vi "启动日志.vi"(8 "error in (no error)":errorcluster, 10 "日志信息":string, 11 "Slave ID":T1=enum."氨氮") -> (0 "error out":errorcluster)   [LabVIEW 2016, in "质控单元V1.lvlib"]
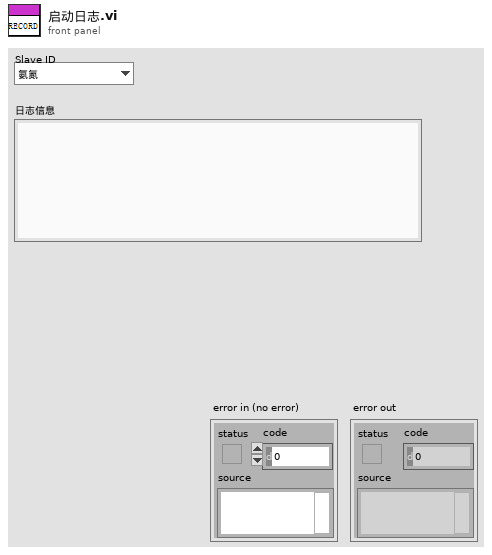
[diagram p1: front panel]
types:
  T1 = typedef "质控单元V1.lvlib/质控slave id.ctl" = enum16{"null", "氨氮", "总磷", "CODMn", "CODCr", "总氮"}
  T2 = typedef "操作日志字段定义.ctl" = cluster{"时间":timestamp, "参数":string, "日志信息":string, "流程参数":string}
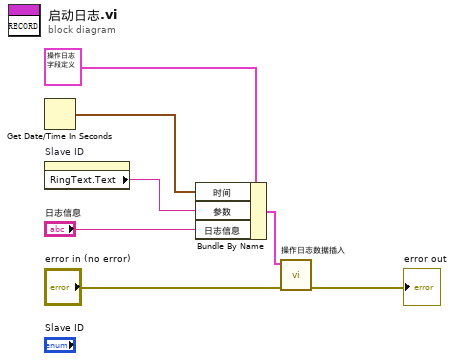
[diagram p0: block diagram]
diagram:
  n1 = Get Date/Time In Seconds() -> (seconds since 1Jan1904=w6:timestamp)
  n2 = property on="Slave ID" class="Enum (严格)"() -> ("RingText.Text"=w5:string)  [unwired: 2 in, 2 out]
  n3 = Bundle By Name(cluster=T2 {"时间"=timestamp(0 s since 1904-01-01), "参数"="水样测试", "日志信息"="N", "流程参数"=""} ("data"), "时间"=w6, "参数"=w5, "日志信息"="日志信息") -> (w3:T2)
  n4 = call "操作日志数据插入.vi"("data"=w3, "错误输入（无错误）"="error in (no error)") -> ("错误输出"=→"error out":errorcluster)  [unwired: 8 in]
